vi "Get Activation Level.vi"() -> (0 "Valid Professional Version":bool)   [LabVIEW 2013, in "VITesterUtilities.lvlib"]
uses:
  Libraries/VITesterUtilities.lvlib
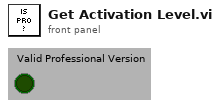
[diagram p1: front panel]
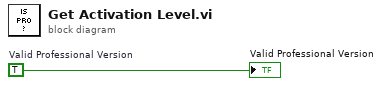
[diagram p0: block diagram]
diagram:
  w1 = TRUE  # Valid Professional Version
  "Valid Professional Version" <- w1
